vi "FPGA_SystemERRWrongVersion.vi"(2 "Revision":u32 format="%.0x", 3 "Version":u16 format="%x") -> (0 "error out":errorcluster)   [LabVIEW 2017]
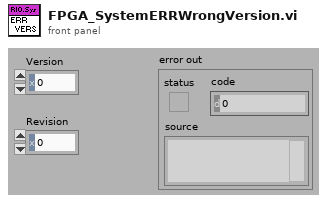
[diagram p1: front panel]
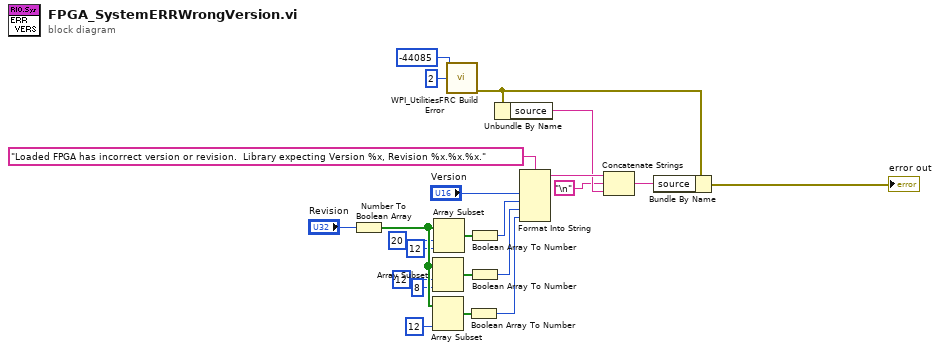
[diagram p0: block diagram]
diagram:
  n1 = Number To Boolean Array(number="Revision") -> (Boolean array=w18:bool[])
  n2 = Array Subset(array=w18, index=12, length=8) -> (w15:bool[])
  n3 = Array Subset(array=w18, length=12) -> (w16:bool[])  [unwired: 1 in]
  n4 = Array Subset(array=w18, index=20, length=12) -> (w17:bool[])
  n5 = call <vilib>:"WPI_UtilitiesFRC Build Error.vi"("error code"=-44085 ("code"), "chain levels to remove (1)"=2) -> ("error out"=w4:errorcluster)  [unwired: 3 in, 10 out]
  n6 = Boolean Array To Number(Boolean array=w16) -> (number=w8:u32)
  n7 = Boolean Array To Number(Boolean array=w17) -> (number=w9:u32)
  n8 = Boolean Array To Number(Boolean array=w15) -> (number=w7:u32)
  n9 = Unbundle By Name(w4) -> ("source"=w2:string)
  n10 = Format Into String(format string="Loaded FPGA has incorrect version or revision.  Library expecting Version %x, Revision %x.%x.%x.", "Version", w9, w7, w8) -> (resulting string=w21:string)  [unwired: 2 in, 1 out]
  n11 = Concatenate Strings(w21, "\n", w2) -> (w3:string)
  n12 = Bundle By Name(cluster=w4, "source"=w3) -> (→"error out":errorcluster)
